vi "WS1021 demo run init.vi"(7 "VNA ports":bool[](array[boolean])=[FALSE, FALSE, TRUE, TRUE], 9 "De-embedding files in":path[](array[path]), 10 "Toggle 8.lvclass in":refnum<class "Toggle 8.lvclass">, 11 "Vector Network Analyzer.lvclass in":refnum<class "Vector Network Analyzer.lvclass">) -> (1 "De-embedding files":path[](array[path]), 2 "Toggle 8.lvclass":refnum<class "Toggle 8.lvclass">, 3 "Vector Network Analyzer.lvclass":refnum<class "Vector Network Analyzer.lvclass">)   [LabVIEW 2020]
uses:
  Instruments/Vector Network Analyzer/Vector Network Analyzer.lvclass
  Devices/Toggle 8/Toggle 8.lvclass
  Devices/Controls/Register to Write.ctl
  Instruments/Vector Network Analyzer/Controls/S parm format enum.ctl
  <vilib>/addons/HF Network Analysis/Support VIs/Read SnP File (SnP).vi
  Devices/PIC-device/PIC-Device.lvclass
  <vilib>/addons/HF Network Analysis/NI_HFNetworkAnalysis.lvlib
panel:
  in  "S parameter":T1(ring)
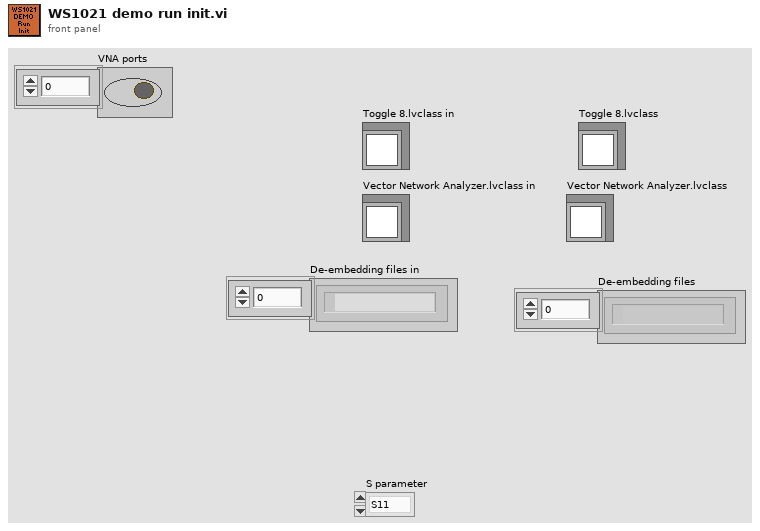
[diagram p1: front panel]
types:
  T1 = enum16{"S11", "S21", "S31", "S41", "S22", "S12", "S32", "S42", "S33", "S13", "S23", "S43", "S44", "S14", "S24", "S34"}
  T2 = typedef "Vector Network Analyzer.lvclass/S parm format enum.ctl" = enum16{"Mag dB", "Mag", "Phase", "Smith", "Real", "Imag", "Group Delay", "SWR"}
  T3 = typedef "PIC-Device.lvclass/Register to Write.ctl" = cluster{"Register":u32, "Value":u32, "Dev Address":u32, "Physical Adress":u32}
  T4 = cluster{"OTP Values string 2":string, "Charge Pump values":enum16{"CP 24V", "CP 26V", "CP 28V", "CP 30V", "CP 31V", "CP 32V", "CP 33V", "CP 34V", "CP 35V", "CP 36V", "CP 37V", "CP 38V", "CP 39V", "CP 40V", "CP 41V", "CP 42V", "CP 43V", "CP 44V", "CP 45V", "CP 46V", "CP 47V", "CP 48V", "CP 49V", "CP 50V", "CP 51V", "CP 52V", "CP 53V", "CP 54V", "CP 56V", "CP 58V", "CP 60V", "CP 62V"}[], "Charge Pump":T3[], "Control individual beams":bool, "OTP/beam values":dbl[], "Capa settings":T3[], "OTP Values string":string}[]
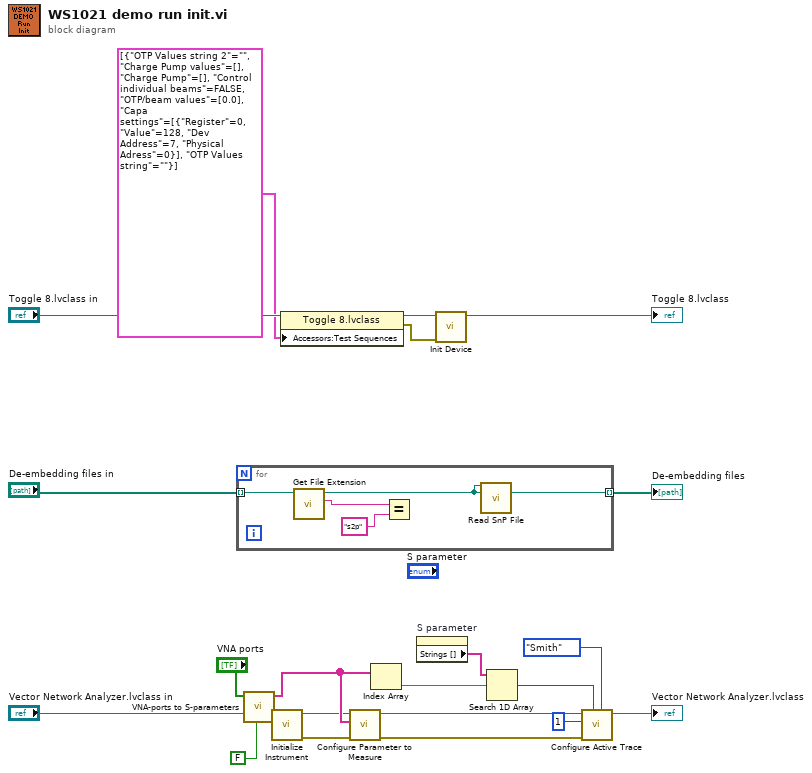
[diagram p0: block diagram]
diagram:
  n1 = for {
    tunnel: "De-embedding files in" -> [w25] mode=indexing
    tunnel: [w22] -> w18 mode=indexing
    n2 = call <vilib>:"Get File Extension.vi"("file"=w25) -> ("lowercase file extension"=w24:string, "dup file"=w22:path)  [unwired: 6 in, 3 out]
    n3 = Equal?(x=w24, y="s2p" ("lowercase file extension")) -> ()  [unwired: 1 out]
    n4 = call-poly <vilib>:"Read SnP File.vi"("SnP File Path"=w22) -> ()  [unwired: 11 in, 4 out]
  }
  "De-embedding files" <- w18
  n5 = call "VNA-ports to S-parameters.vi"("VNA ports"="VNA ports") -> ("Sparameters (string)"=w6:string[])  [unwired: 6 in, 4 out]
  n6 = call-dynamic "Initialize Instrument.vi"("Reset"=FALSE, "Instrument in"="Vector Network Analyzer.lvclass in") -> ("error out"=w2:errorcluster, "Instrument out"=w4:refnum<class "Vector Network Analyzer.lvclass">)  [unwired: 8 in]
  n7 = property class="Toggle 8.lvclass"(reference="Toggle 8.lvclass in", "Accessors:Test Sequences"=T4 [{"OTP Values string 2"="", "Charge Pump values"=[], "Charge Pump"=[], "Control individual beams"=FALSE, "OTP/beam values"=[0.0], "Capa settings"=[{"Register"=0, "Value"=128, "Dev Address"=7, "Physical Adress"=0}], "OTP Values string"=""}] ("Test Sequences")) -> (reference out=w16:refnum<class "Toggle 8.lvclass">, error out=w14:errorcluster)  [unwired: 1 in]
  n8 = call-dynamic "Configure Parameter to Measure.vi"("error in (no error)"=w2, "Sparameters (string)"=w6, "Vector Network Analyzer in"=w4) -> ("error out"=w13:errorcluster, "Vector Network Analyzer out"=w12:refnum<class "Vector Network Analyzer.lvclass">)  [unwired: 7 in]
  n9 = Index Array(array=w6) -> (element=w8:string)  [unwired: 1 in]
  n10 = property on="S parameter" class="Enum (strict)"() -> ("Strings []"=w9:string[])  [unwired: 2 in, 2 out]
  n11 = call-dynamic "Init Device.vi"("error in (no error)"=w14, "Toggle 8 in"=w16) -> ("Toggle 8 out"=→"Toggle 8.lvclass":refnum<class "Toggle 8.lvclass">)  [unwired: 8 in, 1 out]
  n12 = Search 1D Array(1D array=w9, element=w8) -> (index of element=w7:i32)  [unwired: 1 in]
  n13 = call-dynamic "Configure Active Trace.vi"("Format"=S_parm_format_enum."Smith", "S parameter"=w7, "error in (no error)"=w13, "Active Trace"=u8 1, "Vector Network Analyzer in"=w12) -> ("Vector Network Analyzer out"=→"Vector Network Analyzer.lvclass":refnum<class "Vector Network Analyzer.lvclass">)  [unwired: 5 in, 1 out]
